vi "Get Available Configurations.vi"(8 "error in (no error)":errorcluster, 11 "Config in":refnum<class "Config.lvclass">) -> (0 "error out":errorcluster, 2 "Configuration names":string[](array[string]), 3 "Config out":refnum<class "Config.lvclass">)   [LabVIEW 2026, in "TALOS.lvlib" / "Classes.lvlib" / "Config.lvclass"]
uses:
  Config.lvclass
  Config.lvclass/Config.ctl
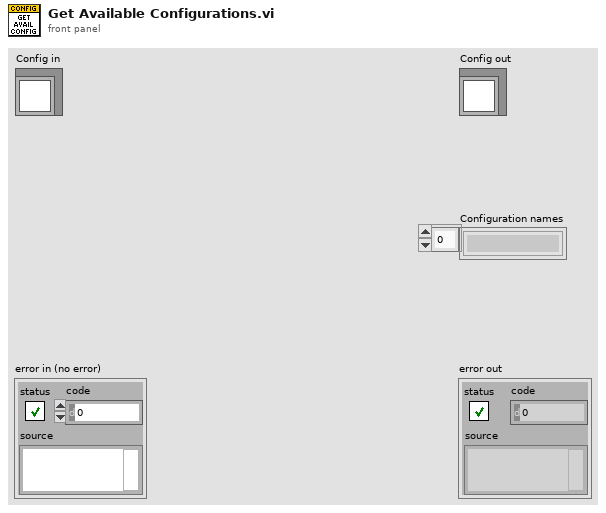
[diagram p1: front panel]
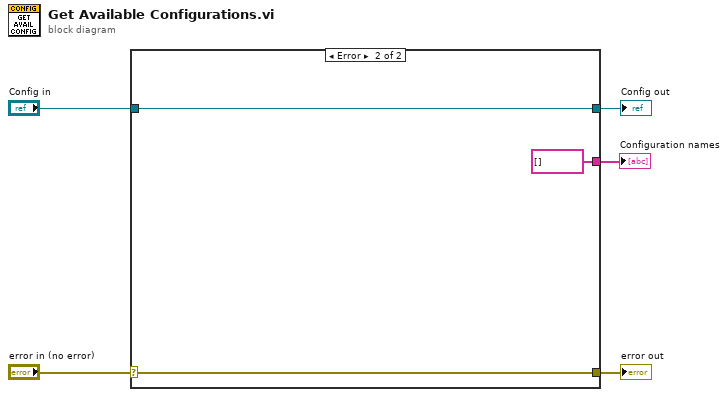
[diagram p0: block diagram]
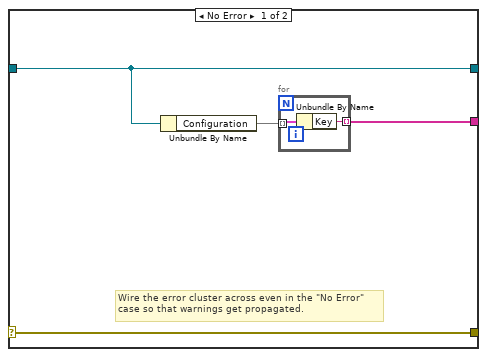
[diagram p2: hidden frame]
diagram:
  n1 = case shown="Error" "error in (no error)" {
    selector: "error in (no error)" -> [w9 w14]
    tunnel: [w9 w14] -> w4
    tunnel: [w8 w13] -> w2
    tunnel: "Config in" -> [w8 w13]
    tunnel: [w6 string[] []] -> w1
    frame No Error {
      # "Wire the error cluster across even in the \"No Error\"\ncase so that warnings get propagated."
      n2 = Unbundle By Name(w8) -> ("Configuration"=w7:map{string, map{string, string}})
      n3 = for {
        tunnel: w7 -> [w11] mode=indexing
        tunnel: [w10] -> w6 mode=indexing
        n4 = Unbundle By Name(w11) -> ("Key"=w10:string)
      }
    }
    frame Error {
    }
  }
  "error out" <- w4
  "Config out" <- w2
  "Configuration names" <- w1
